vi "Motion@AddMotor__Parameter.vi"(1 "ParamterIn":string) -> (0 "ParamterOut":string)   [LabVIEW 2020]
uses:
  MainFrame/Global.vi
panel:
  out "Example Setting:":string
  in  "Driver":string(combo)
  in  "Parameter":string(combo)
  in  "MotorName":string(combo)
  in  "Confirm":bool
  # "Motor@AddMotor $Motor,$Driver,$ParameterS"
  # "CKDAX:                      COM=,ID=\nMISEXRS:                  COM=,ID=\nIAIPCON:                   COM=,ID=\nMITMRJE:                  COM=,ID=\nORARD:                     COM=,ID=\nAMONET1240:            RING=,ID=,BPS={20M,10M,5M,2.5M}  \nAMONET1240X3:        RING=,ID=,BPS={20M,10M,5M,2.5M}  \nAMONET1240X1:        RING=,ID=,BPS={20M,10M,5M,2.5M},AXIS={X,Y,Z,U}\nADLINK8164               CARD=,ID= \nEPSONLS3:                 IP=,PORT=,PASSWD="
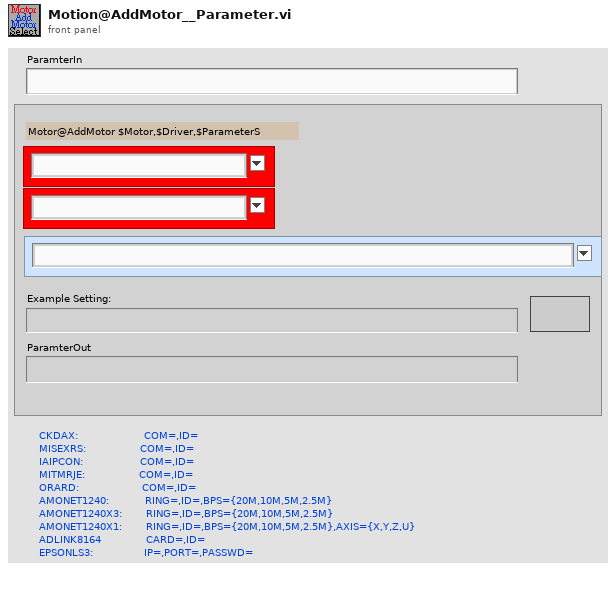
[diagram p1: front panel]
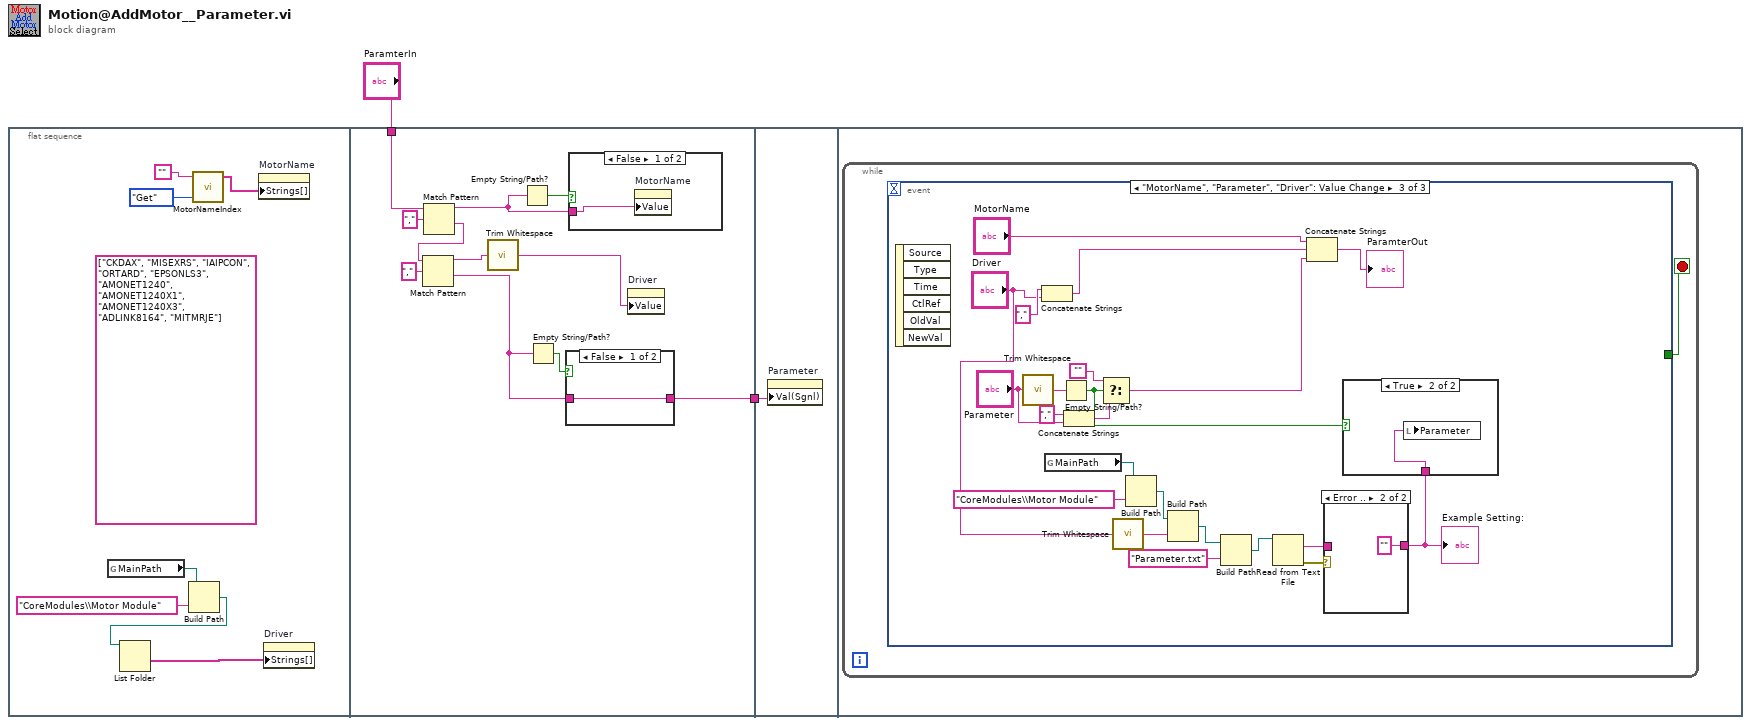
[diagram p0: block diagram]
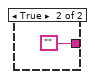
[diagram p2: hidden frame]
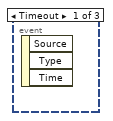
[diagram p4: hidden frame]
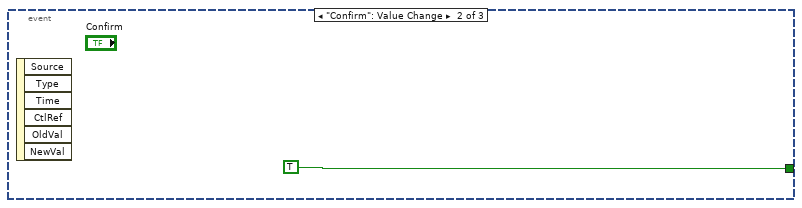
[diagram p5: hidden frame]
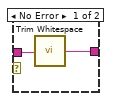
[diagram p7: hidden frame]
diagram:
  n1 = flat-sequence {
    tunnel: "ParamterIn" -> [w17]
    tunnel: [w18] -> w1
    tunnel: w1 -> [w24]
    frame #0 {
      (unwired) string[] ["CKDAX", "MISEXRS", "IAIPCON", "ORTARD", "EPSONLS3", "AMONET1240", "AMONET1240X1", "AMONET1240X3", "ADLINK8164", "MITMRJE"] ("Strings []")
      n2 = global read "Global.vi" "MainPath"() -> (w6:path)
      n3 = Build Path(base path=w6, name or relative path="CoreModules\\Motor Module") -> (appended path=w4:path)
      n4 = List Folder(path=w4) -> (folder names=w3:string[])  [unwired: 3 in, 3 out]
      n5 = call "MotorNameIndex.vi"("OP"=enum16{"Get", "Update", "Init"}."Get", "MotorName"="") -> ("MotorList"=w7:string[])  [unwired: 1 in, 2 out]
      n6 = property on="MotorName" class="CmbBox"("Strings[]"=w7) -> ()  [unwired: 2 in, 2 out]
      n7 = property on="Driver" class="CmbBox"("Strings[]"=w3) -> ()  [unwired: 2 in, 2 out]
    }
    frame #1 {
      n8 = Match Pattern(string=w17, regular expression="," ("search string")) -> (before substring=w15:string, after substring=w13:string)  [unwired: 1 in, 2 out]
      n9 = Match Pattern(string=w13, regular expression="," ("search string")) -> (before substring=w11:string, after substring=w12:string)  [unwired: 1 in, 2 out]
      n10 = call <vilib>:"Trim Whitespace.vi"("string"=w11) -> ("trimmed string"=w10:string)  [unwired: 1 in]
      n11 = Empty String/Path?(string/path=w15) -> (empty?=w20:bool)
      n12 = Empty String/Path?(string/path=w12) -> (empty?=w19:bool)
      n13 = case shown="False" w19 {
        tunnel: [w21 ""] -> w18
        tunnel: w12 -> [w21 _]
        frame False {
        }
        frame True {
        }
      }
      n14 = case shown="False" w20 {
        tunnel: w15 -> [w23 _]
        frame False {
          n15 = property on="MotorName" class="CmbBox"("Value"=w23) -> ()  [unwired: 2 in, 2 out]
        }
        frame True {
        }
      }
      n16 = property on="Driver" class="CmbBox"("Value"=w10) -> ()  [unwired: 2 in, 2 out]
    }
    frame #2 {
      n17 = property on="Parameter" class="CmbBox"("Val(Sgnl)"=w24) -> ()  [unwired: 2 in, 2 out]
    }
    frame #3 {
      n18 = while {
        stop <- w25 stop-if-true
        n19 = event shown="[2] \"MotorName\", \"Parameter\", \"Driver\": Value Change" {
          selector: _ -> [_ _ _]
          dyn-events: _ -> [_ _ _]
          timeout: _ -> [_ _ _]
          tunnel: [_ TRUE _] -> w25
          event Timeout {
            n20 = event-data() -> ()  [unwired: 1 in, 3 out]
          }
          event "Confirm": Value Change {
            n21 = event-data() -> ()  [unwired: 1 in, 6 out]
          }
          event "MotorName", "Parameter", "Driver": Value Change {
            n22 = event-data() -> ()  [unwired: 1 in, 6 out]
            n23 = call <vilib>:"Trim Whitespace.vi"("string"="Parameter") -> ("trimmed string"=w44:string)  [unwired: 1 in]
            n24 = Concatenate Strings(",", "Driver") -> (w41:string)
            n25 = global read "Global.vi" "MainPath"() -> (w37:path)
            n26 = Empty String/Path?(string/path=w44) -> (empty?=w28:bool)
            n27 = Concatenate Strings("," ("string"), "Parameter") -> (w46:string)
            n28 = Select(t="", s=w28, f=w46) -> (s? t:f=w40:string)
            n29 = call <vilib>:"Trim Whitespace.vi"("string"="Driver") -> ("trimmed string"=w35:string)  [unwired: 1 in]
            n30 = Build Path(base path=w37, name or relative path="CoreModules\\Motor Module") -> (appended path=w36:path)
            n31 = Build Path(base path=w36, name or relative path=w35) -> (appended path=w33:path)
            n32 = Build Path(base path=w33, name or relative path="Parameter.txt") -> (appended path=w31:path)
            n33 = Read from Text File(file (use dialog)=w31) -> (text=w29:string, error out=w30:errorcluster)  [unwired: 3 in, 2 out]
            n34 = Concatenate Strings("MotorName", w41, w40) -> (→"ParamterOut":string)
            n35 = case shown="Error .." w30 {
              tunnel: w29 -> [w51 _]
              tunnel: [w50 "" ("trimmed string")] -> w27
              frame No Error {
                n36 = call <vilib>:"Trim Whitespace.vi"("string"=w51) -> ("trimmed string"=w50:string)  [unwired: 1 in]
              }
              frame Error {
              }
            }
            "Example Setting:" <- w27
            n37 = case shown="True" w28 {
              tunnel: w27 -> [_ w49]
              frame False {
              }
              frame True {
                n38 = local write "Parameter"(w49) -> ()
              }
            }
          }
        }
      }
    }
  }
